vi "CMD Execute Graphviz.vi"(8 "error in":errorcluster, 10 "Img Type":T1, 11 "Dot File":path) -> (0 "error out":errorcluster, 3 "Dependency Plot":picture)   [LabVIEW 2020, in "SimpleDependencyInspector.lvlib"]
uses:
  Libraries/SimpleDependencyInspector/SimpleDependencyInspector.lvlib
  Libraries/SimpleDependencyInspector/Image Type--enum.ctl
  <vilib>/Platform/browser.llb/Open URL in Default Browser (path).vi
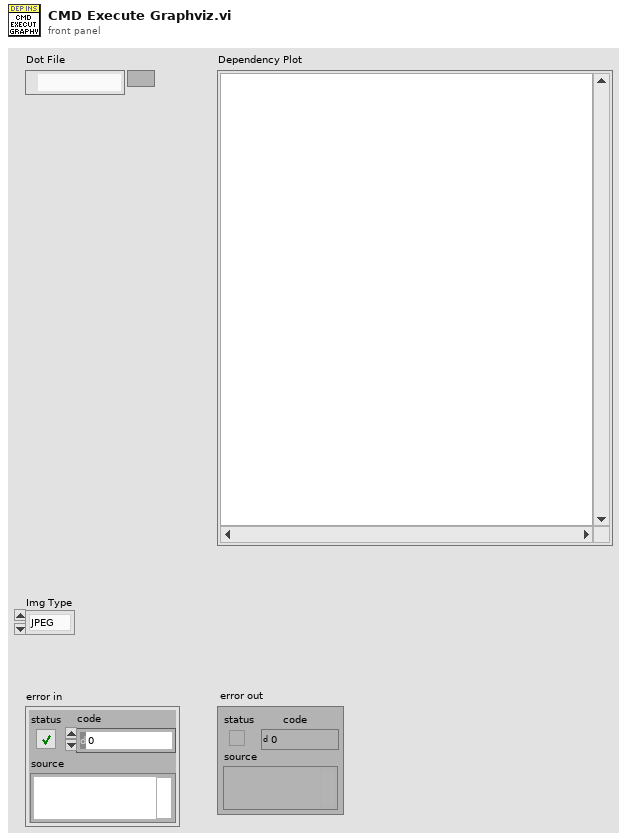
[diagram p1: front panel]
types:
  T1 = typedef "SimpleDependencyInspector.lvlib/Image Type--enum.ctl" = enum16{"JPEG", "PNG", "BMP", "SVG"}
  T2 = typedef "imagedata.ctl" = cluster{"image type":i32, "image depth":i32, "image":u8[], "mask":u8[], "colors":u32[], "Rectangle":cluster{"left":i16, "top":i16, "right":i16, "bottom":i16}}
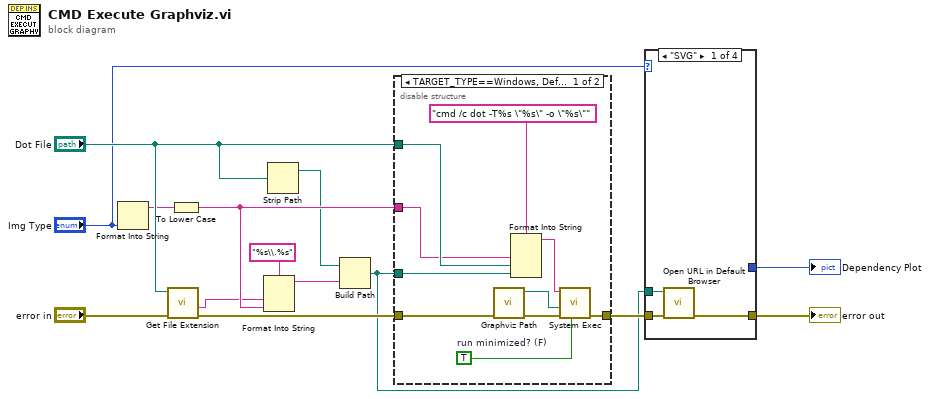
[diagram p0: block diagram]
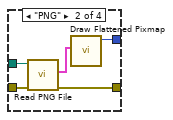
[diagram p2: hidden frame]
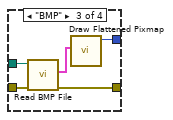
[diagram p3: hidden frame]
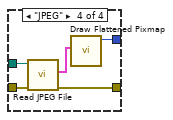
[diagram p4: hidden frame]
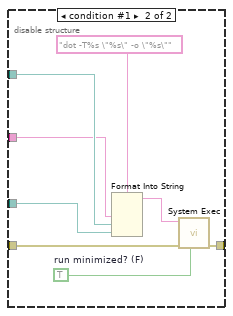
[diagram p5: hidden frame]
diagram:
  n1 = Format Into String("Img Type") -> (resulting string=w9:string)  [unwired: 3 in, 1 out]
  n2 = call <vilib>:"Get File Extension.vi"("error in (no error)"="error in", "file"="Dot File") -> ("error out"=w11:errorcluster, "filename without extension"=w4:string)  [unwired: 5 in, 3 out]
  n3 = To Lower Case(string=w9) -> (all lower case string=w8:string)
  n4 = Format Into String(format string="%s\\.%s", w4, w8) -> (resulting string=w5:string)  [unwired: 2 in, 1 out]
  n5 = Strip Path(path="Dot File") -> (stripped path=w3:path)  [unwired: 1 out]
  n6 = Build Path(base path=w3, name or relative path=w5) -> (appended path=w1:path)
  n7 = disable-structure shown="TARGET_TYPE==Windows, Default" {
    disable-tunnel: [w23 w32] -> w13
    disable-tunnel: "Dot File" -> [w17 w27]
    disable-tunnel: w8 -> [w16 w26]
    disable-tunnel: w1 -> [w15 w25]
    disable-tunnel: w11 -> [w22 w31]
    frame condition #0 (active) {
      w21 = TRUE  # run minimized? (F)
      n8 = call "Graphviz Path.vi"("error in"=w22) -> ("error out"=w24:errorcluster, "Graphviz Path"=w18:path)  [unwired: 9 in]
      n9 = Format Into String(format string="cmd /c dot -T%s \"%s\" -o \"%s\"" ("command line"), w16, w17, w15) -> (resulting string=w19:string)  [unwired: 2 in, 1 out]
      n10 = call <vilib>:"System Exec.vi"("run minimized? (F)"=w21, "error in (no error)"=w24, "working directory"=w18, "command line"=w19) -> ("error out"=w23:errorcluster)  [unwired: 4 in, 3 out]
    }
    frame condition #1 {
      w30 = TRUE  # run minimized? (F)
      n11 = Format Into String(format string="dot -T%s \"%s\" -o \"%s\"" ("command line"), w26, w27, w25) -> (resulting string=w28:string)  [unwired: 2 in, 1 out]
      n12 = call <vilib>:"System Exec.vi"("run minimized? (F)"=w30, "error in (no error)"=w31, "command line"=w28) -> ("error out"=w32:errorcluster)  [unwired: 5 in, 3 out]
    }
  }
  n13 = case shown="\"SVG\"" "Img Type" {
    tunnel: w13 -> [w35 w40 w45 w50]
    tunnel: [w34 w39 w44 w49] -> w12
    tunnel: w1 -> [w33 w37 w42 w47]
    tunnel: [_ w36 w41 w46] -> w7
    frame "SVG" {
      n14 = call-poly <vilib>:"Open URL in Default Browser.vi"("error in (no error)"=w35, "path"=w33) -> ("error out"=w34:errorcluster)  [unwired: 4 in, 1 out]
    }
    frame "PNG" {
      n15 = call <vilib>:"Read PNG File.vi"("error in (no error)"=w40, "path to PNG file"=w37) -> ("error out"=w39:errorcluster, "image data"=w38:T2)  [unwired: 7 in, 1 out]
      n16 = call <vilib>:"Draw Flattened Pixmap.vi"("image data"=w38) -> ("new picture"=w36:picture)  [unwired: 8 in]
    }
    frame "BMP" {
      n17 = call <vilib>:"Read BMP File.vi"("error in (no error)"=w45, "path to BMP file"=w42) -> ("error out"=w44:errorcluster, "image data"=w43:T2)  [unwired: 7 in, 1 out]
      n18 = call <vilib>:"Draw Flattened Pixmap.vi"("image data"=w43) -> ("new picture"=w41:picture)  [unwired: 8 in]
    }
    frame "JPEG" {
      n19 = call <vilib>:"Read JPEG File.vi"("error in (no error)"=w50, "path to JPEG file"=w47) -> ("error out"=w49:errorcluster, "image data"=w48:T2)  [unwired: 7 in, 1 out]
      n20 = call <vilib>:"Draw Flattened Pixmap.vi"("image data"=w48) -> ("new picture"=w46:picture)  [unwired: 8 in]
    }
  }
  "error out" <- w12
  "Dependency Plot" <- w7
